vi "Individual LBCB Readings.vi"() -> ()   [LabVIEW 2009]
uses:
  lib/Launcher/Launcher Actions.ctl
  lib/Launcher/NoPanelAppTypes.ctl
  lib/Data Access Objects/Metadata/DAO Actions.ctl
panel:
  out "LBCB 1 Data":dbl[][](array[numeric])
  out "LBCB 2 Data":dbl[][](array[numeric])
  out "DOF Labels 2":string[](array[string])=["Dx", "Dy", "Dz", "Rx", "Ry", "Rz"]
  out "DOF Labels":string[](array[string])=["Dx", "Dy", "Dz", "Rx", "Ry", "Rz"]
  in  "Ok":bool
  # "Forces"
  # "Displacements"
  # "Commands"
  # "LBCB 1"
  # "LBCB 2"
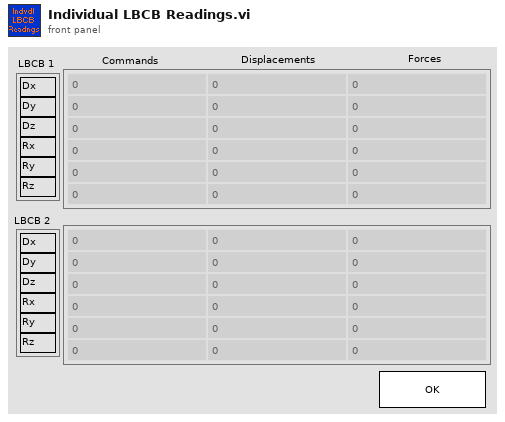
[diagram p1: front panel]
types:
  T1 = typedef "NoPanelAppTypes.ctl" = enum16{"NTCP Socket", "Data Archiving", "DAQ Link", "Control Loops", "Cmd Disp Diffs", "Individual Readings", "Limits", "Increment Limits"}
  T2 = typedef "Launcher Actions.ctl" = enum16{"Launch", "Stop All", "Stop", "Kill", "Running?", "Init"}
  T3 = typedef "DAO Actions.ctl" = enum16{"Init", "Get", "Set"}
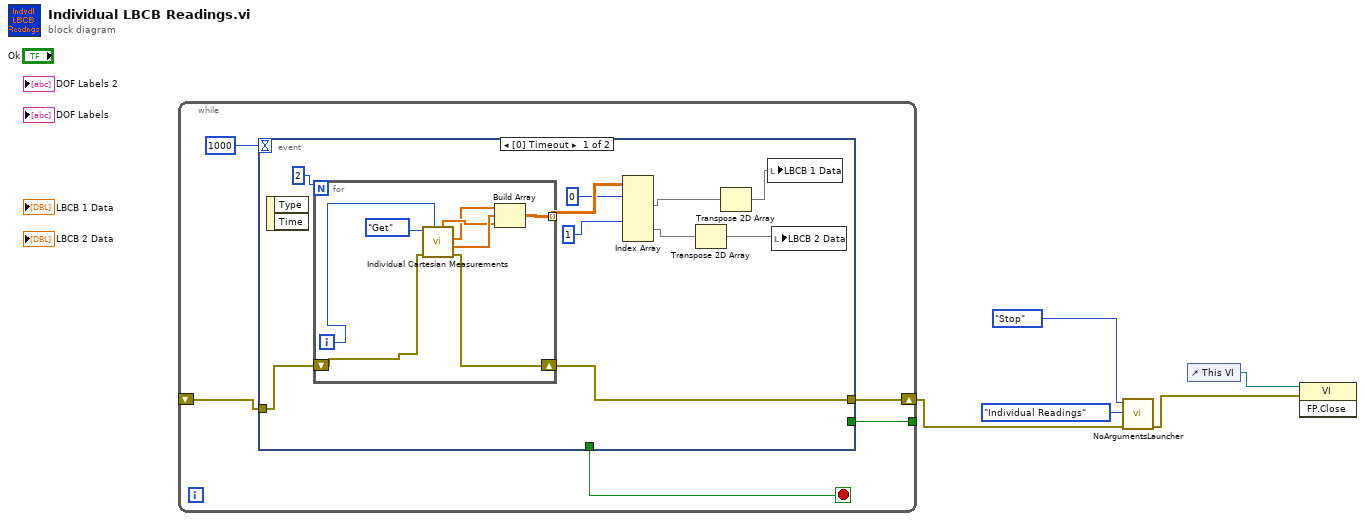
[diagram p0: block diagram]
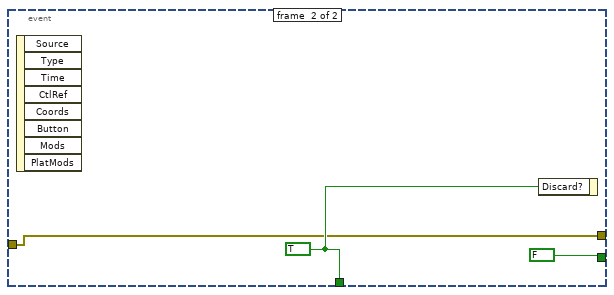
[diagram p2: hidden frame]
diagram:
  n1 = while {
    tunnel: [w8] -> _
    shift-right: [w6] -> w5
    shift-left: _ -> [w7]
    stop <- w9 stop-if-true
    n2 = event shown="[0] Timeout" {
      selector: _ -> [_ _]
      dyn-events: _ -> [_ _]
      timeout: 1000 -> [_ _]
      tunnel: [_ w30] -> w9
      tunnel: [_ FALSE] -> w8
      tunnel: w7 -> [w20 w29]
      tunnel: [w19 w29] -> w6
      event #0 {
        n3 = event-data() -> ()  [unwired: 3 out]
        n4 = for {
          N: 2 -> [_]
          shift-right: [w23] -> w19
          shift-left: w20 -> [w24]
          tunnel: [w25] -> w17 mode=indexing
          i -> [w22]
          n5 = call "Individual Cartesian Measurements.vi"("LBCB Number"=w22, "error in (no error)"=w24, "DAO Actions"=DAO_Actions."Get") -> ("error out"=w23:errorcluster, "Displacements Out"=w27:dbl[], "Commands Out"=w21:dbl[], "Forces Out"=w26:dbl[])  [unwired: 5 in]
          n6 = Build Array(w21, w27, w26) -> (w25:dbl[][])
        }
        n7 = Index Array(array=w17, index (dim 0) #1=0 ("index (page)"), index (dim 0) #2=1 ("index (page)")) -> (element #1=w16:dbl[][], element #2=w15:dbl[][])  [unwired: 4 in]
        n8 = Transpose 2D Array(2D array=w15) -> (transposed array=w11:dbl[][])
        n9 = Transpose 2D Array(2D array=w16) -> (transposed array=w12:dbl[][])
        n10 = local write "LBCB 1 Data"(w12) -> ()
        n11 = local write "LBCB 2 Data"(w11) -> ()
      }
      event #1 {
        w30 = TRUE
        n12 = event-data() -> ()  [unwired: 9 out]
        n13 = event-data("Discard?"=w30) -> ()  [unwired: 1 in, 1 out]
      }
    }
  }
  n14 = call "NoArgumentsLauncher.vi"("error in (no error)"=w5, "Application"=NoPanelAppTypes."Individual Readings", "Application Launcher Actions"=Launcher_Actions."Stop") -> ("error out"=w1:errorcluster)  [unwired: 8 out]
  n15 = control-ref of="This VI"() -> (w4:refnum<vi>)
  n16 = invoke class="VI" method="FP.Close"(reference=w4, error in=w1) -> ()  [unwired: 1 in, 3 out]
